vi "GV DO1.vi"() -> ()   [LabVIEW 2017]
panel:
  out "DO1":bool
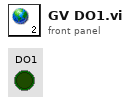
[diagram p1: front panel]
diagram:
